vi "Table_ResetTableCell.vi"(8 "error in (no error)":errorcluster, 11 "Listbox Ref":refnum<vi>) -> (0 "error out":errorcluster, 3 "Listbox Ref":refnum<vi>)   [LabVIEW 2012, in "TableSupportLib.lvlib"]
uses:
  TableSupportLib.lvlib
  <vilib>/Utility/miscctls.llb/LVRowAndColumnTypeDef.ctl
  <vilib>/Utility/miscctls.llb/LVRowAndColumnUnsignedTypeDef.ctl
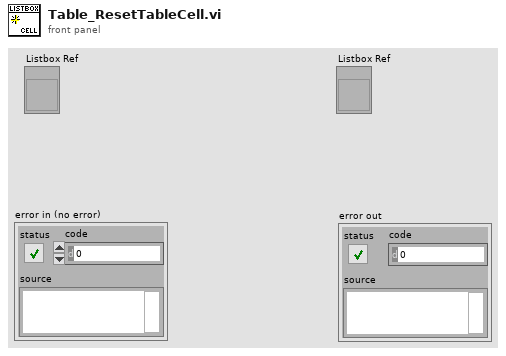
[diagram p1: front panel]
types:
  T1 = typedef "LVRowAndColumnUnsignedTypeDef.ctl" = cluster{"Row":u32, "Column":u32}
  T2 = typedef "LVRowAndColumnTypeDef.ctl" = cluster{"Row":i32, "Column":i32}
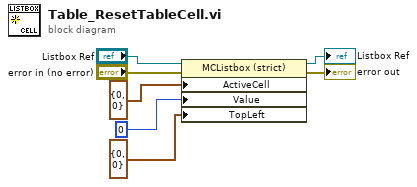
[diagram p0: block diagram]
diagram:
  n1 = property class="MCListbox (strict)"(reference="Listbox Ref", error in="error in (no error)", "ActiveCell"=T2 {"Row"=0, "Column"=0} ("Active Cell:Active Cell"), "Value"=0, "TopLeft"=T1 {"Row"=0, "Column"=0} ("Top Left Visible Cell")) -> (reference out=→"Listbox Ref":refnum<vi>, error out=→"error out":errorcluster)
